vi "trial one - Seprate loops.vi"() -> ()   [LabVIEW 2018]
uses:
  <vilib>/MakerHub/Xbox-One-Controller/Private/Type Defs/Indicators/All Axis Data.ctl
  <vilib>/MakerHub/Xbox-One-Controller/Private/Type Defs/Indicators/DPad Enum.ctl
  <vilib>/Instr/_visa.llb/VISA Configure Serial Port (Instr).vi
  <vilib>/MakerHub/Xbox-One-Controller/Public/Open First Controller.vi
  <vilib>/MakerHub/Xbox-One-Controller/LMH-Xbox-One-Controller.lvlib
panel:
  out "element 3":string
  out "element 2":string
  out "element":string
  out "RT Y - axis":string
  out "RT X-axis":string
  out "LT Y- axis":string
  out "Right Stick":cluster{"X Axis":i32, "Y Axis":i32}
  out "Left Stick":cluster{"X Axis":i32, "Y Axis":i32}
  out "Event Log 4":string[](array[string])
  out "All Axis 4":T1
  in  "write buffer":string
  out "byte count":u32
  out "Rx Slave Msg":string
  in  "delay before read (ms)":u32=500
  in  "Write":bool=TRUE
  in  "Read":bool=TRUE
  in  "stop":bool
  in  "flow control (0:none)":u16(ring) items=["None", "XON/XOFF", "RTS/CTS", "XON/XOFF & RTS/CTS", "DTR/DSR", "XON/XOFF & DTR/DSR"]
  in  "stop bits (10: 1 bit)":u16(ring)=10 items=["1.0"=10, "1.5"=15, "2.0"=20]
  in  "parity (0:none)":enum16{"None", "Odd", "Even", "Mark", "Space"}(ring)
  in  "data bits (8)":u16=8 min=5 max=8 step=1
  in  "baud rate (9600)":u32=9600
  in  "VISA resource name":refnum<visa-resource-name>="COM1"
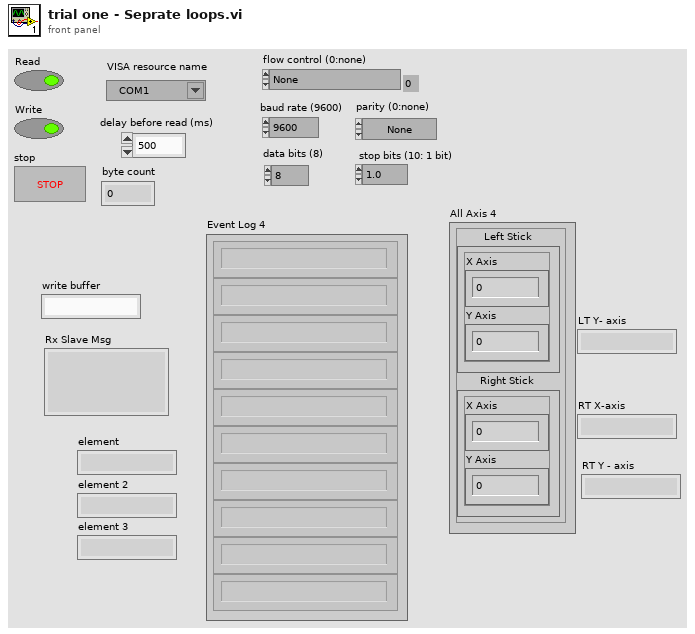
[diagram p1: front panel]
types:
  T1 = typedef "LMH-Xbox-One-Controller.lvlib/All Axis Data.ctl" = cluster{"Left Stick":cluster{"X Axis":i32, "Y Axis":i32}, "Right Stick":cluster{"X Axis":i32, "Y Axis":i32}, "Triggers":i32, "D-Pad":T2}
  T2 = typedef "LMH-Xbox-One-Controller.lvlib/DPad Enum.ctl" = enum16{"Idle", "Up", "Up / Right", "Right", "Down / Right", "Down", "Down / Left", "Left", "Up / Left"}
  T3 = typedef "LMH-Xbox-One-Controller.lvlib/Xbox One Controller Ref.ctl" = cluster{"Controller Ref":refnum<k1>, "Event Refnum":refnum<event-registration>, "Worker Ref":refnum<vi>}
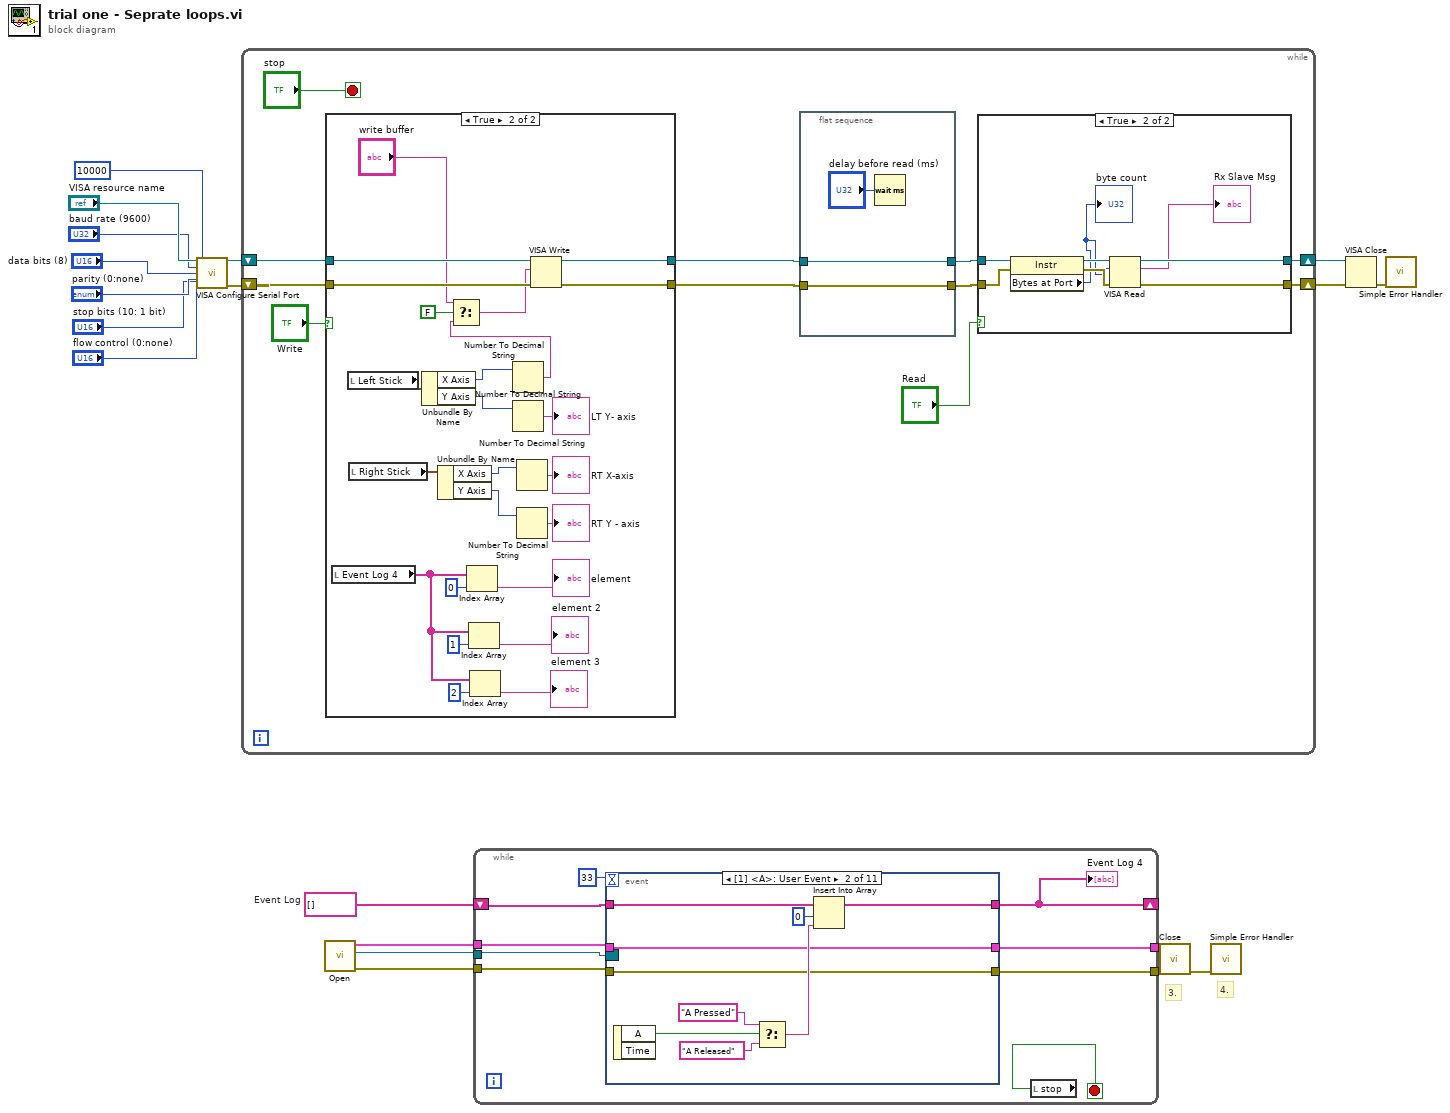
[diagram p0: block diagram]
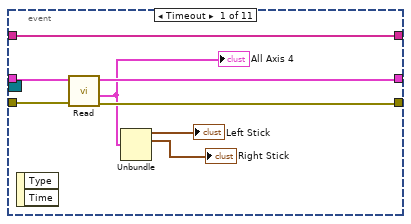
[diagram p2: hidden frame]
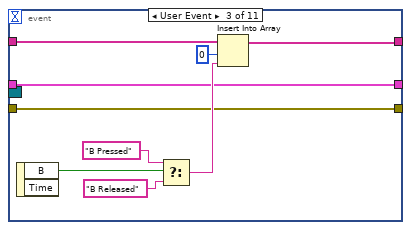
[diagram p3: hidden frame]
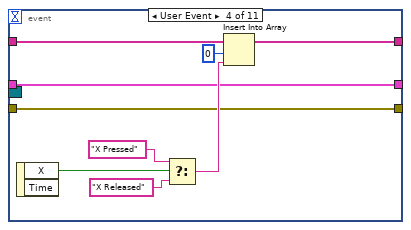
[diagram p4: hidden frame]
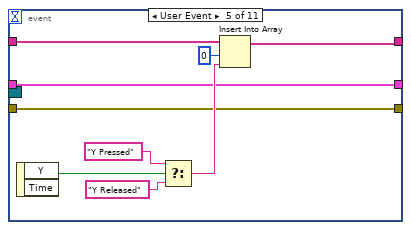
[diagram p5: hidden frame]
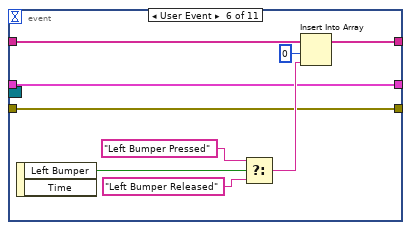
[diagram p6: hidden frame]
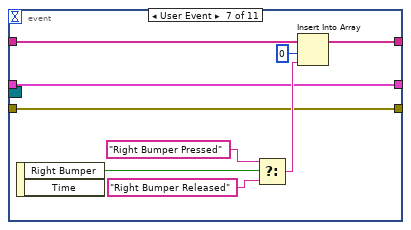
[diagram p7: hidden frame]
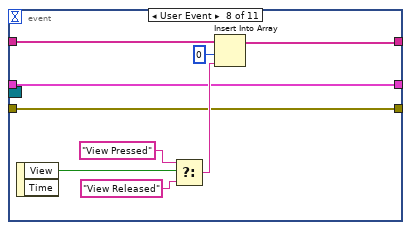
[diagram p8: hidden frame]
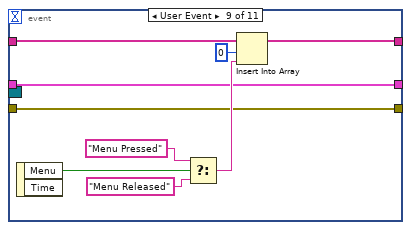
[diagram p9: hidden frame]
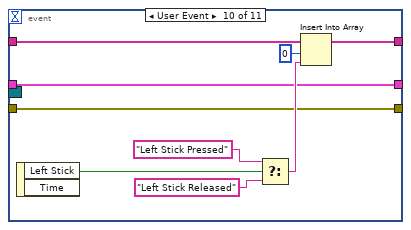
[diagram p10: hidden frame]
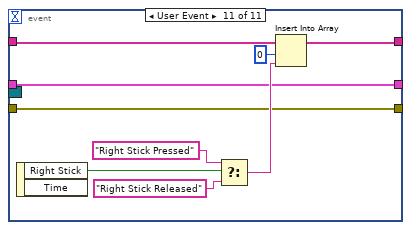
[diagram p11: hidden frame]
diagram:
  w6 = string[] []  # Event Log
  # "4."
  # "3."
  n1 = call-poly "VISA Configure Serial Port"("VISA resource name"="VISA resource name", "timeout (10sec)"=u32 10000, "baud rate (9600)"="baud rate (9600)", "data bits (8)"="data bits (8)", "parity (0:none)"="parity (0:none)", "stop bits (10: 1 bit)"="stop bits (10: 1 bit)", "flow control (0:none)"="flow control (0:none)") -> ("VISA resource name out"=w19:refnum<visa-resource-name>, "error out"=w18:errorcluster)  [unwired: 7 in]
  n2 = while {
    shift-right: [w25] -> w17
    shift-left: w19 -> [w23]
    shift-right: [w24] -> w16
    shift-left: w18 -> [w22]
    stop <- "stop" stop-if-true
    n3 = case shown="True" "Write" {
      tunnel: [w45 w69] -> w30
      tunnel: [w44 w68] -> w29
      tunnel: w23 -> [w45 w67]
      tunnel: w22 -> [w44 w66]
      frame False {
      }
      frame True {
        n4 = local read "Event Log 4"() -> (w50:string[])
        n5 = local read "Left Stick"() -> (w62:cluster{"X Axis":i32, "Y Axis":i32})
        n6 = local read "Right Stick"() -> (w58:cluster{"X Axis":i32, "Y Axis":i32})
        n7 = Unbundle By Name(w62) -> ("X Axis"=w61:i32, "Y Axis"=w59:i32)
        n8 = Unbundle By Name(w58) -> ("X Axis"=w57:i32, "Y Axis"=w56:i32)
        n9 = Index Array(array=w50, index=0) -> (element=→"element":string)
        n10 = Index Array(array=w50, index=1) -> (element=→"element 2":string)
        n11 = Index Array(array=w50, index=2) -> (element=→"element 3":string)
        n12 = Number To Decimal String(number=w61) -> (decimal integer string=w60:string)  [unwired: 1 in]
        n13 = Select(t="write buffer", s=FALSE, f=w60) -> (s? t:f=w64:string)
        n14 = Number To Decimal String(number=w59) -> (decimal integer string=→"LT Y- axis":string)  [unwired: 1 in]
        n15 = Number To Decimal String(number=w57) -> (decimal integer string=→"RT X-axis":string)  [unwired: 1 in]
        n16 = Number To Decimal String(number=w56) -> (decimal integer string=→"RT Y - axis":string)  [unwired: 1 in]
        n17 = VISA Write(VISA resource name=w67, write buffer=w64, error in (no error)=w66) -> (VISA resource name out=w69:refnum<visa-resource-name>, error out=w68:errorcluster)  [unwired: 1 out]
      }
    }
    n18 = flat-sequence {
      tunnel: w30 -> [w33]
      tunnel: w29 -> [w32]
      tunnel: [w33] -> w28
      tunnel: [w32] -> w27
      frame #0 {
        n19 = Wait (ms)(milliseconds to wait="delay before read (ms)") -> ()  [unwired: 1 out]
      }
    }
    n20 = case shown="True" "Read" {
      tunnel: [w35 w43] -> w25
      tunnel: [w34 w42] -> w24
      tunnel: w28 -> [w35 w41]
      tunnel: w27 -> [w34 w40]
      frame False {
      }
      frame True {
        n21 = property class="Instr"(reference=w41, error in=w40) -> (reference out=w39:refnum<visa-resource-name>, error out=w38:errorcluster, "Bytes at Port"=w37:u32)
        "byte count" <- w37
        n22 = VISA Read(VISA resource name=w39, byte count=w37, error in (no error)=w38) -> (VISA resource name out=w43:refnum<visa-resource-name>, read buffer=→"Rx Slave Msg":string, error out=w42:errorcluster)  [unwired: 1 out]
      }
    }
  }
  n23 = call-poly <vilib>:"Open.vi"() -> ("Error Out"=w3:errorcluster, "Event Refnum"=w4:refnum<event-registration>, "Xbox One Controller"=w5:T3)  [unwired: 9 in]
  n24 = while {
    shift-right: [w77] -> _
    shift-left: w6 -> [w76]
    tunnel: w5 -> [w75]
    tunnel: w4 -> [w74]
    tunnel: w3 -> [w73]
    tunnel: [w72] -> w2
    tunnel: [w71] -> w1
    stop <- w70 stop-if-true
    n25 = event shown="[1] <A>: User Event" {
      selector: w74 -> [_ _ _ _ _ _ _ _ _ _ _]
      dyn-events: _ -> [_ _ _ _ _ _ _ _ _ _ _]
      timeout: 33 -> [_ _ _ _ _ _ _ _ _ _ _]
      tunnel: w75 -> [w86 w89 w97 w109 w119 w128 w134 w144 w151 w161 w171]
      tunnel: w73 -> [w85 w88 w98 w110 w118 w123 w135 w145 w152 w160 w170]
      tunnel: [w82 w88 w98 w110 w118 w123 w135 w145 w152 w160 w170] -> w71
      tunnel: [w84 w89 w97 w109 w119 w128 w134 w144 w151 w161 w171] -> w72
      tunnel: w76 -> [w83 w95 w100 w108 w116 w127 w136 w143 w154 w163 w172]
      tunnel: [w83 w90 w99 w107 w115 w126 w137 w142 w155 w164 w173] -> w77
      event Timeout {
        n26 = event-data() -> ()  [unwired: 1 in, 2 out]
        n27 = call <vilib>:"Read.vi"("Error In"=w85, "Xbox One Controller Ref"=w86) -> ("Error Out"=w82:errorcluster, "All Axis"=w81:T1, "Xbox One Controller Ref"=w84:T3)  [unwired: 6 in, 1 out]
        "All Axis 4" <- w81
        n28 = Unbundle(w81) -> ("Left Stick"=→"Left Stick":cluster{"X Axis":i32, "Y Axis":i32}, "Right Stick"=→"Right Stick":cluster{"X Axis":i32, "Y Axis":i32})  [unwired: 2 out]
      }
      event User Event {
        n29 = event-data() -> ("A"=w94:bool)  [unwired: 1 in, 1 out]
        n30 = Select(t="A Pressed" ("String"), s=w94, f="A Released" ("String")) -> (s? t:f=w91:string)
        n31 = Insert Into Array(array=w95, index=0, new element=w91) -> (w90:string[])
      }
      event User Event {
        n32 = event-data() -> ("B"=w101:bool)  [unwired: 1 in, 1 out]
        n33 = Select(t="B Pressed" ("String"), s=w101, f="B Released" ("String")) -> (s? t:f=w102:string)
        n34 = Insert Into Array(array=w100, index=0, new element=w102) -> (w99:string[])
      }
      event User Event {
        n35 = event-data() -> ("X"=w106:bool)  [unwired: 1 in, 1 out]
        n36 = Select(t="X Pressed" ("String"), s=w106, f="X Released" ("String")) -> (s? t:f=w111:string)
        n37 = Insert Into Array(array=w108, index=0, new element=w111) -> (w107:string[])
      }
      event User Event {
        n38 = event-data() -> ("Y"=w117:bool)  [unwired: 1 in, 1 out]
        n39 = Select(t="Y Pressed" ("String"), s=w117, f="Y Released" ("String")) -> (s? t:f=w120:string)
        n40 = Insert Into Array(array=w116, index=0, new element=w120) -> (w115:string[])
      }
      event User Event {
        n41 = event-data() -> ("Left Bumper"=w125:bool)  [unwired: 1 in, 1 out]
        n42 = Select(t="Left Bumper Pressed" ("String"), s=w125, f="Left Bumper Released" ("String")) -> (s? t:f=w129:string)
        n43 = Insert Into Array(array=w127, index=0, new element=w129) -> (w126:string[])
      }
      event User Event {
        n44 = event-data() -> ("Right Bumper"=w133:bool)  [unwired: 1 in, 1 out]
        n45 = Select(t="Right Bumper Pressed" ("String"), s=w133, f="Right Bumper Released" ("String")) -> (s? t:f=w138:string)
        n46 = Insert Into Array(array=w136, index=0, new element=w138) -> (w137:string[])
      }
      event User Event {
        n47 = event-data() -> ("View"=w146:bool)  [unwired: 1 in, 1 out]
        n48 = Select(t="View Pressed" ("String"), s=w146, f="View Released" ("String")) -> (s? t:f=w147:string)
        n49 = Insert Into Array(array=w143, index=0, new element=w147) -> (w142:string[])
      }
      event User Event {
        n50 = event-data() -> ("Menu"=w153:bool)  [unwired: 1 in, 1 out]
        n51 = Select(t="Menu Pressed" ("String"), s=w153, f="Menu Released" ("String")) -> (s? t:f=w156:string)
        n52 = Insert Into Array(array=w154, index=0, new element=w156) -> (w155:string[])
      }
      event User Event {
        n53 = event-data() -> ("Left Stick"=w162:bool)  [unwired: 1 in, 1 out]
        n54 = Select(t="Left Stick Pressed" ("String"), s=w162, f="Left Stick Released" ("String")) -> (s? t:f=w165:string)
        n55 = Insert Into Array(array=w163, index=0, new element=w165) -> (w164:string[])
      }
      event User Event {
        n56 = event-data() -> ("Right Stick"=w169:bool)  [unwired: 1 in, 1 out]
        n57 = Select(t="Right Stick Pressed" ("String"), s=w169, f="Right Stick Released" ("String")) -> (s? t:f=w174:string)
        n58 = Insert Into Array(array=w172, index=0, new element=w174) -> (w173:string[])
      }
    }
    "Event Log 4" <- w77
    n59 = local read "stop"() -> (w70:bool)
  }
  n60 = call <vilib>:"Close.vi"("Error In"=w1, "Xbox One Controller Ref"=w2) -> ("Error Out"=w7:errorcluster)  [unwired: 9 in]
  n61 = call <vilib>:"Simple Error Handler.vi"("error in (no error)"=w7) -> ()  [unwired: 4 in, 5 out]
  n62 = VISA Close(VISA resource name=w17, error in (no error)=w16) -> (error out=w8:errorcluster)
  n63 = call <vilib>:"Simple Error Handler.vi"("error in (no error)"=w8) -> ()  [unwired: 4 in, 5 out]
